vi "C4LV_searchDevices.vi"(0 "c4if Arr in":refnum<k24>[](array[refnum]), 11 "error in (no error)":errorcluster) -> (4 "c4if Arr out":refnum<k24>[](array[refnum]), 6 "devName out":string[](array[string]), 15 "error out":errorcluster)   [LabVIEW 2015, in "libC4HdlLV.lvlib"]
uses:
  libC4HdlLV.lvlib
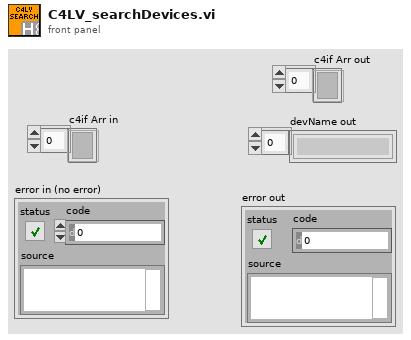
[diagram p1: front panel]
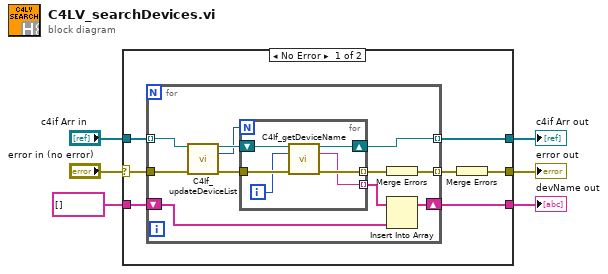
[diagram p0: block diagram]
diagram:
  n1 = case shown="No Error" "error in (no error)" {
    selector: "error in (no error)" -> [w7 w33]
    tunnel: "c4if Arr in" -> [w13 w32]
    tunnel: [w12 w32] -> w1
    tunnel: [w10 w33] -> w6
    tunnel: [w9 w31] -> w5
    tunnel: string[] [] -> [w8 w31]
    frame No Error {
      n2 = for {
        tunnel: w13 -> [w16] mode=indexing
        tunnel: w7 -> [w18]
        tunnel: [w24] -> w12 mode=indexing
        tunnel: [w22] -> w11 mode=indexing
        shift-right: [w20] -> w9
        shift-left: w8 -> [w19]
        n3 = call "C4If_updateDeviceList.vi"("c4if in"=w16, "error in (no error)"=w18) -> ("c4if out"=w15:refnum<k24>, "nofDev out"=w14:i64, "error out"=w17:errorcluster)  [unwired: 11 in]
        n4 = for {
          N: w14 -> [_]
          tunnel: w17 -> [w30]
          tunnel: [w25] -> w21 mode=indexing
          tunnel: [w29] -> w23 mode=indexing
          shift-right: [w27] -> w24
          shift-left: w15 -> [w28]
          i -> [w26]
          n5 = call "C4If_getDeviceName.vi"("c4if in"=w28, "devNo in"=w26, "error in (no error)"=w30) -> ("c4if out"=w27:refnum<k24>, "device name out"=w25:string, "error out"=w29:errorcluster)  [unwired: 10 in]
        }
        n6 = Merge Errors(w23) -> (w22:errorcluster)
        n7 = Insert Into Array(array=w21, new element=w19) -> (w20:string[])  [unwired: 1 in]
      }
      n8 = Merge Errors(w11) -> (w10:errorcluster)
    }
    frame Error {
    }
  }
  "error out" <- w6
  "devName out" <- w5
  "c4if Arr out" <- w1
